vi "SetFocus.vi"(8 "error in (no error)":errorcluster, 11 "hWnd (NULL)":T1) -> (0 "error out":errorcluster, 3 "dup hWnd":T1)   [LabVIEW 2011]
doc: "SetFocus\nThe SetFocus function sets the keyboard focus to the specified window. The window must be associated with the calling thread's message queue. \n\nHWND SetFocus(\n HWND hWnd // handle to window to receive focus\n);\n \nParameters\nhWnd \nHandle to the window that will receive the keyboard input. If this parameter is NULL, keystrokes are ignored. \nReturn Values\nIf the function succeeds, the return value is the handle to the window that previously had the keyboard focus. If the hWnd parameter is invalid or the window is not associated with the calling thread's message queue, the return value is NULL. To get extended error information, callGetLastError.\n\nRemarks\nThe SetFocus function sends a WM_KILLFOCUS message to the window that loses the keyboard focus and a WM_SETFOCUS message to the window that receives the keyboard focus. It also activates either the window that receives the focus or the parent of the window that receives the focus. \n\nIf a window is active but does not have the focus, any key pressed will produce the WM_SYSCHAR, WM_SYSKEYDOWN, or WM_SYSKEYUP message. If the VK_MENU key is also pressed, the lParam parameter of the message will have bit 30 set. Otherwise, the messages produced do not have this bit set. \n\nBy using the AttachThreadInput function, a thread can attach its input processing to another thread. This allows a thread to call SetFocus to set the keyboard focus to a window associated with another thread's message queue. \n\nWindows CE: Do not use the SetFocus function to set the keyboard focus to a window associated with another thread's message queue. There is one exception. If a window on one thread is the child of the window on the other thread, or if the windows are siblings of the same parent, the thread associated with one window can set the focus to the other window even though it belongs to a different thread. In this case, there is no need to call AttachThreadInput first."
uses:
  hWnd.ctl
  user32.dll
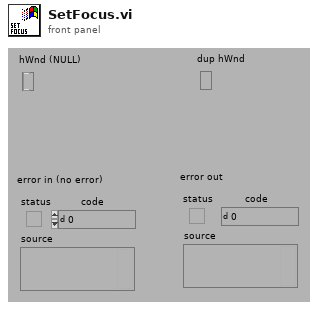
[diagram p1: front panel]
types:
  T1 = typedef "hWnd.ctl" = refnum<k1>
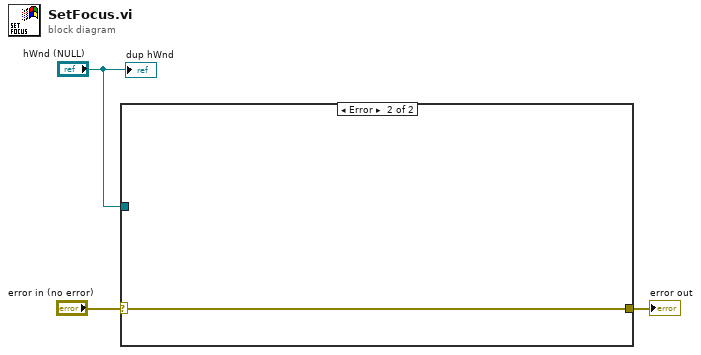
[diagram p0: block diagram]
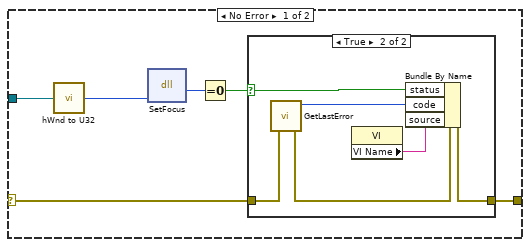
[diagram p2: hidden frame]
diagram:
  n1 = case shown="Error" "error in (no error)" {
    selector: "error in (no error)" -> [w5 w17]
    tunnel: [w6 w17] -> w3
    tunnel: "hWnd (NULL)" -> [w8 _]
    frame No Error {
      n2 = call "hWnd to U32.vi"("hWnd"=w8) -> ("hWnd"=w7:u32)  [unwired: 4 out]
      n3 = dll-call lib="user32.dll" fn="SetFocus"("hWnd"=w7) -> ("hWnd"=w9:u32)  [unwired: 4 in, 2 out]
      n4 = Equal To 0?(x=w9) -> (x = 0?=w4:bool)
      n5 = case shown="True" w4 {
        selector: w4 -> [_ w11]
        tunnel: w5 -> [w10 w15]
        tunnel: [w10 w16] -> w6
        frame False {
        }
        frame True {
          n6 = call "GetLastError.vi"("error in (no error)"=w15) -> ("error out"=w14:errorcluster, "CODE"=w13:i32)  [unwired: 5 out]
          n7 = property class="VI"() -> ("VI Name"=w12:string)  [unwired: 2 in, 2 out]
          n8 = Bundle By Name(cluster=w14, "status"=w11, "code"=w13, "source"=w12) -> (w16:errorcluster)
        }
      }
    }
    frame Error {
    }
  }
  "error out" <- w3
  "dup hWnd" <- "hWnd (NULL)"
